vi "FPGA Communication.vi"(6 "Stop Button":bool, 8 "error in":errorcluster, 10 "Count(uSec)":u32, 11 "Samples per Channel":u32) -> (0 "error out":errorcluster, 1 "Timed Out?":bool)   [LabVIEW 2021]
uses:
  Typedefs/Q Action.ctl
  Typedefs/Message FPGA.ctl
  <vilib>/rvi/interface/RandomDataEmulation/nirviRandomDataOpen.vi
  <vilib>/rvi/interface/common/niFpgaCacheSessionInfoDynamic.vi
  <vilib>/Utility/error.llb/Error Cluster From Error Code.vi
  <vilib>/rvi/errors/niLvFpgaAdjustHostInterfaceError.vi
  <vilib>/FPGAPlugInAG/Dynamic/niLvFpga_Run_Dynamic.vi
  <vilib>/FPGAPlugInAG/Dynamic/niLvFpga_Close_Dynamic.vi
  <vilib>/rvi/interface/nirviOpenFPGA/nirviOpenFPGA.xnode
  FPGA Target/FPGA Main.vi
  <vilib>/rvi/interface/nirviMethod/nirviMethod.xnode
  <vilib>/rvi/interface/nirviReadWriteControl/nirviReadWriteControl.xnode
  <vilib>/rvi/interface/nirviCloseFPGA/nirviCloseFPGA.xnode
  <vilib>/rvi/errors/niLvFpgaMergeErrorWithErrorCode.vi
  <vilib>/rvi/interface/Simulation/niFpgaSimulationCallBeginRW.vi
  <vilib>/FPGAPlugInAG/Dynamic/niLvFpga_ReadFifo_Dynamic.vi
  <vilib>/FPGAPlugInAG/Dynamic/niLvFpga_StartFifo_Dynamic.vi
  NiFpgaLv.dll
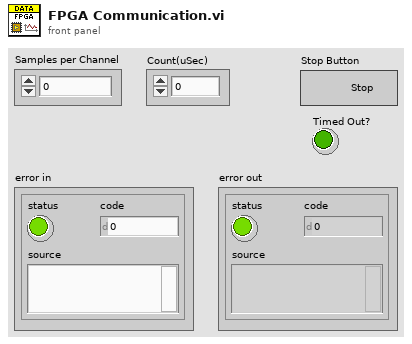
[diagram p1: front panel]
types:
  T1 = typedef "Q Action.ctl" = enum16{"Obtain Queue", "Enqueue", "Dequeue", "Close"}
  T2 = typedef "Message FPGA.ctl" = cluster{"Channel 1 Data (L1 U)":dbl[], "Channel 2 Data (L1 I)":dbl[], "Channel 3 Data (L2 U)":dbl[], "Channel 4 Data (L2 I)":dbl[], "Channel 5 Data (L3 U)":dbl[], "Channel 6 Data (L3 I)":dbl[]}
  T3 = enum16{"open", "open or create", "create or replace", "create", "open (read-only)"}
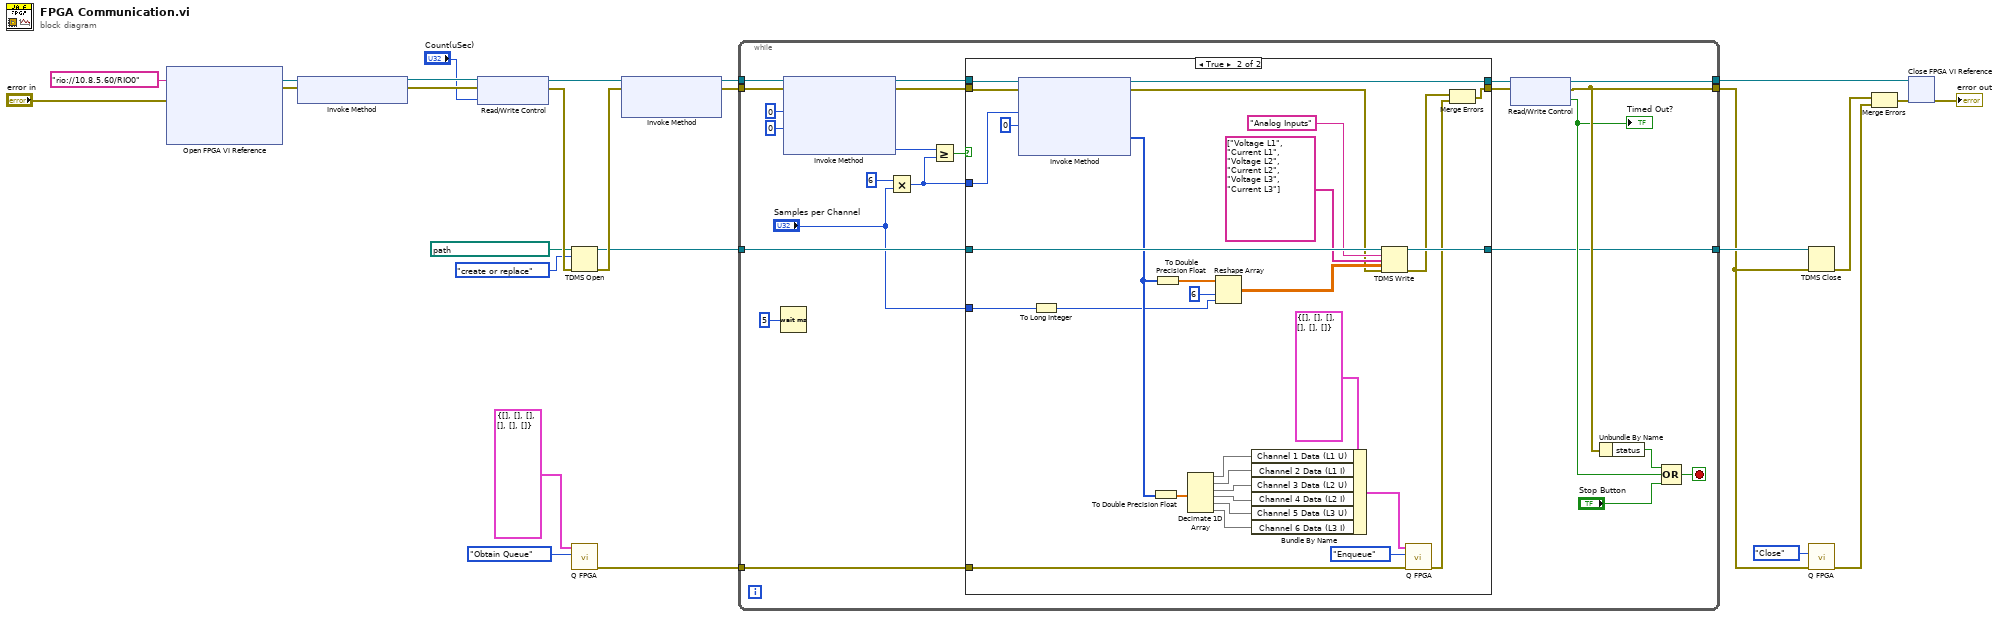
[diagram p0: block diagram]
diagram:
  n1 = xnode "Open FPGA VI Reference"("error in"="error in", "resource name"=tag "rio://10.8.5.60/RIO0") -> ("FPGA VI Reference Out"=w21:refnum<k20>, "error out"=w20:errorcluster)
  n2 = xnode "Invoke Method"("FPGA VI Reference In"=w21, "error in"=w20) -> ("FPGA VI Reference Out"=w19:refnum<k20>, "error out"=w18:errorcluster)
  n3 = xnode "Read/Write Control"("FPGA VI Reference In"=w19, "error in"=w18, "Count(uSec)"="Count(uSec)") -> ("FPGA VI Reference Out"=w25:refnum<k20>, "error out"=w15:errorcluster)
  n4 = TDMS Open(8:w15, 10:T3."create or replace" ("operation (0:open)"), 11:path "F:/AGH - Inżynieria Biomedyczna (I i II stopień)/PRACA MAGISTERSKA/FPGA Project - POWER METER/Data/analog_input.tdms" ("file path")) -> (0:w14:errorcluster, 3:w10:refnum<k34>)  [unwired: 4 in]
  n5 = call "Q FPGA.vi"("Action"=Q_Action."Obtain Queue", "Message FPGA in"=T2 {"Channel 1 Data (L1 U)"=[], "Channel 2 Data (L1 I)"=[], "Channel 3 Data (L2 U)"=[], "Channel 4 Data (L2 I)"=[], "Channel 5 Data (L3 U)"=[], "Channel 6 Data (L3 I)"=[]}) -> ("Error out"=w6:errorcluster)  [unwired: 7 in, 2 out]
  n6 = xnode "Invoke Method"("FPGA VI Reference In"=w25, "error in"=w14) -> ("FPGA VI Reference Out"=w24:refnum<k20>, "error out"=w23:errorcluster)  [unwired: 1 in]
  n7 = while {
    tunnel: w24 -> [w36]
    tunnel: w23 -> [w35]
    tunnel: [w46] -> w26
    tunnel: [w45] -> w5
    tunnel: w10 -> [w43]
    tunnel: [w41] -> w9
    tunnel: w6 -> [w28]
    stop <- w49 stop-if-true
    n8 = Wait (ms)(milliseconds to wait=u32 5 ("millisecond multiple")) -> ()  [unwired: 1 out]
    n9 = xnode "Invoke Method"("FPGA VI Reference In"=w36, "error in"=w35, "Number of Elements"=u32 0, "Timeout (ms)"=0) -> ("FPGA VI Reference Out"=w33:refnum<k20>, "error out"=w42:errorcluster, "Elements Remaining"=w30:u32)  [unwired: 1 out]
    n10 = Multiply(x=u32 6 ("y"), y="Samples per Channel") -> (x*y=w29:u32)
    n11 = Greater Or Equal?(x=w30, y=w29) -> (x >= y?=w31:bool)
    n12 = case shown="True" w31 {
      tunnel: w43 -> [w50 w82]
      tunnel: w42 -> [w51 w76]
      tunnel: [w50 w79] -> w41
      tunnel: [w51 w55] -> w40
      tunnel: w33 -> [w52 w75]
      tunnel: [w52 w74] -> w32
      tunnel: w29 -> [_ w72]
      tunnel: "Samples per Channel" -> [_ w67]
      tunnel: w28 -> [_ w56]
      frame False {
      }
      frame True {
        n13 = xnode "Invoke Method"("FPGA VI Reference In"=w75, "error in"=w76, "Number of Elements"=w72, "Timeout (ms)"=0) -> ("FPGA VI Reference Out"=w74:refnum<k20>, "error out"=w68:errorcluster, "Data"=w70:u32[])  [unwired: 1 out]
        n14 = To Long Integer(number=w67) -> (32bit integer=w66:i32)
        n15 = To Double Precision Float(number=w70) -> (double precision float=w69:dbl[])
        n16 = To Double Precision Float(number=w70) -> (double precision float=w78:dbl[])
        n17 = Decimate 1D Array(w69) -> (w62:dbl[], w61:dbl[], w60:dbl[], w57:dbl[], w58:dbl[], w59:dbl[])
        n18 = Reshape Array(w78, 6 ("dimension size"), w66) -> (w71:dbl[][])
        n19 = Bundle By Name(cluster=T2 {"Channel 1 Data (L1 U)"=[], "Channel 2 Data (L1 I)"=[], "Channel 3 Data (L2 U)"=[], "Channel 4 Data (L2 I)"=[], "Channel 5 Data (L3 U)"=[], "Channel 6 Data (L3 I)"=[]} ("Message FPGA in"), "Channel 1 Data (L1 U)"=w62, "Channel 2 Data (L1 I)"=w61, "Channel 3 Data (L2 U)"=w60, "Channel 4 Data (L2 I)"=w57, "Channel 5 Data (L3 U)"=w58, "Channel 6 Data (L3 I)"=w59) -> (w64:T2)
        n20 = TDMS Write(0:w82, 5:"Analog Inputs" ("group name in (Untitled)"), 7:string[] ["Voltage L1", "Current L1", "Voltage L2", "Current L2", "Voltage L3", "Current L3"] ("channel name(s) in (Untitled)"), 9:w71, 11:w68) -> (4:w79:refnum<k34>, 15:w54:errorcluster)  [unwired: 1 in, 2 out]
        n21 = call "Q FPGA.vi"("Error in"=w56, "Action"=Q_Action."Enqueue", "Message FPGA in"=w64) -> ("Error out"=w53:errorcluster)  [unwired: 6 in, 2 out]
        n22 = Merge Errors(w54, w53) -> (w55:errorcluster)
      }
    }
    n23 = xnode "Read/Write Control"("FPGA VI Reference In"=w32, "error in"=w40) -> ("FPGA VI Reference Out"=w46:refnum<k20>, "error out"=w45:errorcluster, "Overflow?"=w44:bool)
    "Timed Out?" <- w44
    n24 = Unbundle By Name(w45) -> ("status"=w48:bool)
    n25 = Compound Arithmetic op=OR(w48, w44, "Stop Button") -> (w49:bool)
  }
  n26 = TDMS Close(8:w5, 11:w9) -> (0:w2:errorcluster)  [unwired: 1 out]
  n27 = call "Q FPGA.vi"("Error in"=w5, "Action"=Q_Action."Close") -> ("Error out"=w1:errorcluster)  [unwired: 7 in, 2 out]
  n28 = Merge Errors(w2, w1) -> (w3:errorcluster)
  n29 = xnode "Close FPGA VI Reference"("FPGA VI Reference In"=w26, "error in"=w3) -> ("error out"=→"error out":errorcluster)
